vi "SetOperatorMessage.vi"(8 "error in (no error)":errorcluster, 10 "Value":string, 11 "GUI_Handler_Main in":refnum<class "GUI_Handler_Main.lvclass">) -> (0 "error out":errorcluster, 3 "GUI_Handler_Main out":refnum<class "GUI_Handler_Main.lvclass">)   [LabVIEW 2019, in "GUI_Handler_Main.lvclass"]
uses:
  GUI_Handler_Main.lvclass
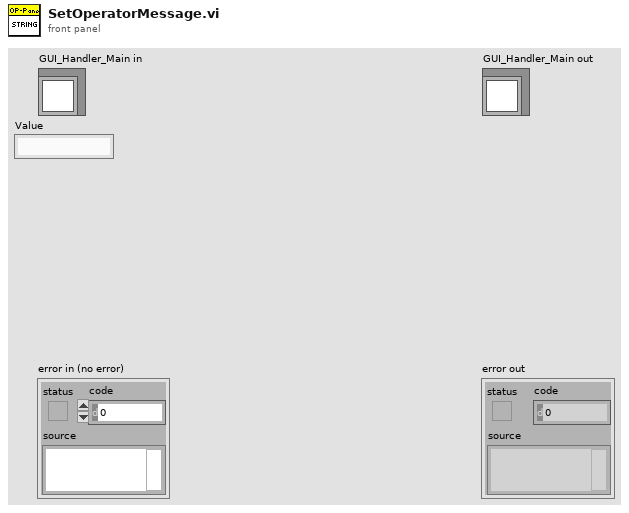
[diagram p1: front panel]
types:
  T1 = cluster{"Operator_Aceept":bool, "Operator_decline ":bool, "User message ":string}
  T2 = cluster{"Start Alt":refnum<vi>, "Stop":refnum<vi>, "Operatør beskeder":refnum<vi>}
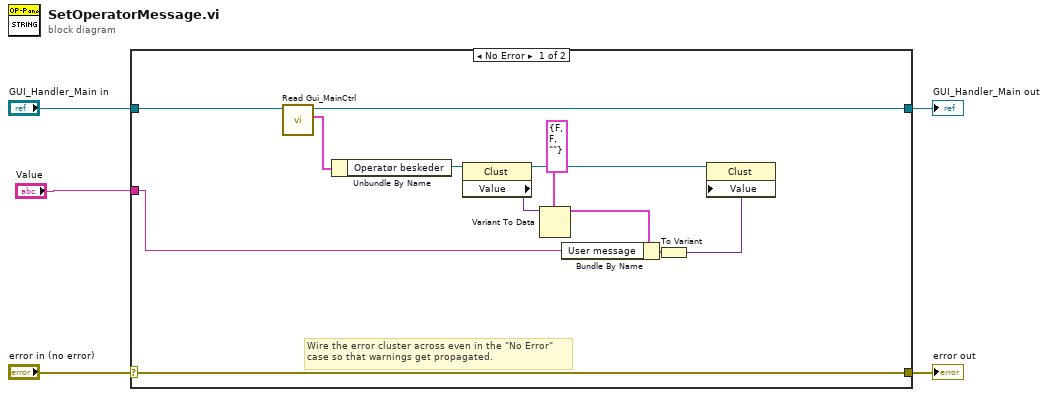
[diagram p0: block diagram]
diagram:
  n1 = case shown="No Error" "error in (no error)" {
    selector: "error in (no error)" -> [w17 w19]
    tunnel: [w17 w19] -> w4
    tunnel: [w15 w18] -> w2
    tunnel: "GUI_Handler_Main in" -> [w16 w18]
    tunnel: "Value" -> [w9 _]
    frame No Error {
      # "Wire the error cluster across even in the \"No Error\"\ncase so that warnings get propagated."
      n2 = call-dynamic "Read Gui_MainCtrl.vi"("GUI_Handler_Main in"=w16) -> ("Gui_MainCtrl"=w14:T2, "GUI_Handler_Main out"=w15:refnum<class "GUI_Handler_Main.lvclass">)  [unwired: 8 in, 1 out]
      n3 = Unbundle By Name(w14) -> ("Operatør beskeder"=w13:refnum<vi>)
      n4 = property class="Clust"(reference=w13) -> (reference out=w6:refnum<vi>, "Value"=w12:variant)  [unwired: 1 in, 1 out]
      n5 = Variant To Data(type=T1 {"Operator_Aceept"=FALSE, "Operator_decline "=FALSE, "User message "=""} ("Operatør beskeder"), Variant=w12) -> (data=w10:T1)  [unwired: 1 in, 1 out]
      n6 = Bundle By Name(cluster=w10, "User message"=w9) -> (w8:T1)
      n7 = To Variant(anything=w8) -> (Variant=w7:variant)
      n8 = property class="Clust"(reference=w6, "Value"=w7) -> ()  [unwired: 1 in, 2 out]
    }
    frame Error {
    }
  }
  "error out" <- w4
  "GUI_Handler_Main out" <- w2
